vi "Robot Global Data.vi"() -> ()   [LabVIEW 2011]
doc: "This global VI can contain as many global variables as you need. Place a control on the panel, give it a good name. To read or write to it from a VI, drag the icon to the diagram of that VI. You can also drag from the project. Click on the node to change which global you access. You shouldn't have multiple locations writing to a global or it will cause a race-condition."
uses:
  <vilib>/Rock Robotics/WPI/Camera/WPI_CameraImageSize.ctl
  <vilib>/Rock Robotics/WPI/Joystick/WPI_JoystickButtonState.ctl
panel:
  out "Ball Switch":bool
  out "Encoder Mean Voltage":dbl
  out "Encoder Voltage":dbl
  in  "Hammer speed setting":dbl
  out "Drive Buttons":T1
  in  "Ball Elevator speed setting":dbl
  in  "Ball Collector speed setting":dbl
  out "Sonar Mean Voltage":dbl
  in  "Shooter Preset 4":dbl=0.9
  in  "Shooter Preset 3":dbl=0.8
  in  "Shooter Preset 2":dbl=0.7
  in  "Shooter Preset 1":dbl=0.6
  in  "Use Shooter Presets":bool=TRUE
  in  "Shooter speed setting":dbl
  out "Sonar Voltage":dbl
  out "global shooting speed  array":cluster{dbl, dbl}[](array[cluster])
  out "Buttons":T1
  in  "LED toggle rate (ms)":u32=20
  in  "image size":T2=enum."320x240"
  in  "Enable Vision":bool=TRUE
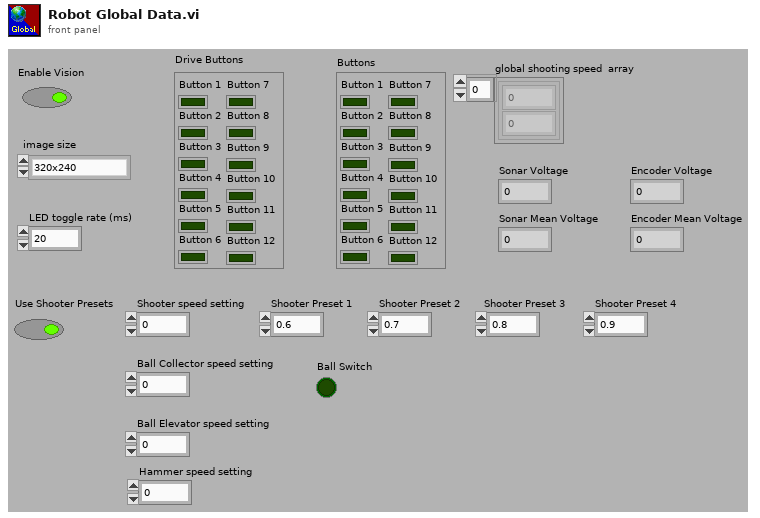
[diagram p1: front panel]
types:
  T1 = typedef "WPI_JoystickButtonState.ctl" = cluster{"Button 1":bool, "Button 2":bool, "Button 3":bool, "Button 4":bool, "Button 5":bool, "Button 6":bool, "Button 7":bool, "Button 8":bool, "Button 9":bool, "Button 10":bool, "Button 11":bool, "Button 12":bool}
  T2 = typedef "WPI_CameraImageSize.ctl" = enum16{"640x480", "320x240", "160x120"}
diagram:
